vi "Socket Read.vi"(8 "error in (no error)":errorcluster, 9 "timeout ms (5000)":i32=5000, 10 "# bytes to read":i32, 11 "WebSocket in":refnum<class "WebSocket.lvclass">) -> (0 "error out":errorcluster, 1 "timed out?":bool, 2 "Read Bytes":u8[](array[numeric]), 3 "WebSocket out":refnum<class "WebSocket.lvclass">)   [LabVIEW 2021, in "WebSockets.lvlib" / "WebSocket.lvclass"]
doc: "Wrapper for the Socket Read function.\nWebSockets 2.0.1.40\nSam Sharp - MediaMongrels Ltd\nCopyright (c) 2019, MediaMongrels Ltd"
uses:
  WebSocket.lvclass
  WebSocket.lvclass/WebSocket.ctl
  Sockets/Socket/Socket.lvclass
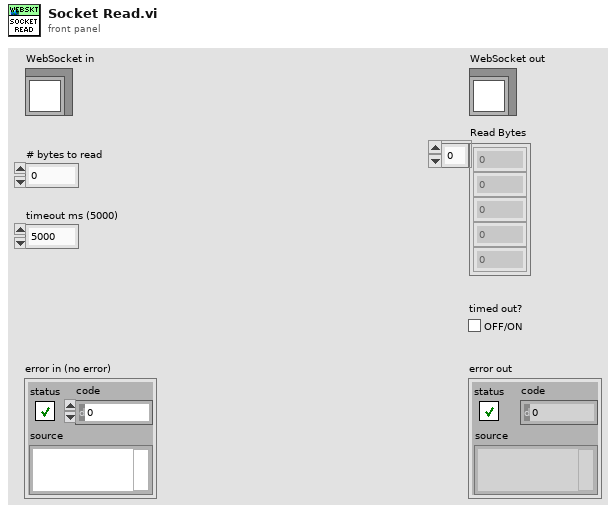
[diagram p1: front panel]
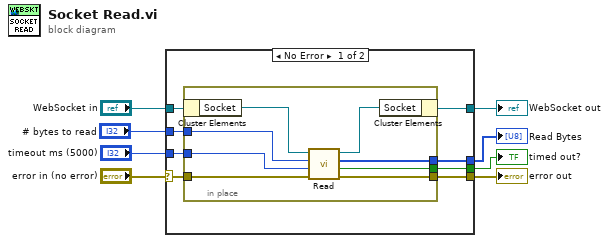
[diagram p0: block diagram]
diagram:
  n1 = case shown="No Error" "error in (no error)" {
    selector: "error in (no error)" -> [w14 w25]
    tunnel: [w12 w26] -> w6
    tunnel: "WebSocket in" -> [w16 w26]
    tunnel: "timeout ms (5000)" -> [w15 _]
    tunnel: [w13 w25] -> w4
    tunnel: [w11 _] -> w3
    tunnel: "# bytes to read" -> [w10 _]
    tunnel: [w9 _] -> w1
    frame No Error {
      n2 = in-place {
        in-place-border: w15 -> [w23]
        in-place-border: w14 -> [w22]
        in-place-border: [w21] -> w13
        in-place-border: [w19] -> w11
        in-place-border: w10 -> [w18]
        in-place-border: [w17] -> w9
        n3 = in-place-cluster #1(w16) -> ("Socket"=w24:refnum<class "Socket.lvclass">)
        n4 = call-dynamic "Read.vi"("error in (no error)"=w22, "timeout ms (25000)"=w23, "# bytes to read"=w18, "Socket in"=w24) -> ("error out"=w21:errorcluster, "timed out?"=w17:bool, "Read Bytes"=w19:u8[], "Socket out"=w20:refnum<class "Socket.lvclass">)  [unwired: 4 in]
        n5 = in-place-cluster #1("Socket"=w20) -> (w12:refnum<class "WebSocket.lvclass">)
      }
    }
    frame Error {
    }
  }
  "error out" <- w4
  "WebSocket out" <- w6
  "Read Bytes" <- w3
  "timed out?" <- w1
